vi "write_bytes.vi"(8 "error in (no error)":errorcluster, 9 "timeout ms (-1)":i32=-1, 10 "data in":string, 11 "TCP Connection in":refnum<class "TCP Connection.lvclass">) -> (0 "error out":errorcluster, 1 "bytes written":i32, 2 "timeout?":bool, 3 "TCP Connection out":refnum<class "TCP Connection.lvclass">)   [LabVIEW 2019, in "TCP Connection.lvclass"]
uses:
  TCP Connection.lvclass
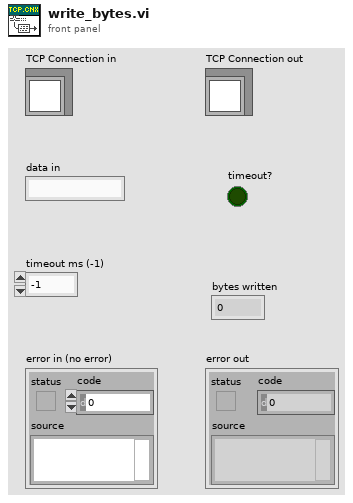
[diagram p1: front panel]
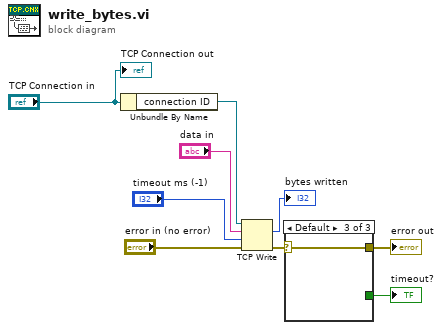
[diagram p0: block diagram]
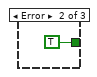
[diagram p3: hidden frame]
diagram:
  n1 = Unbundle By Name("TCP Connection in") -> ("connection ID"=w8:refnum<k5>)
  n2 = TCP Write(connection ID=w8, data in="data in", error in (no error)="error in (no error)", 9:"timeout ms (-1)") -> (bytes written=→"bytes written":i32, error out=w3:errorcluster)  [unwired: 1 out]
  n3 = case shown="Default" w3 {
    selector: w3 -> [w10 _ w12]
    tunnel: [w10 _ w12] -> w2
    tunnel: [_ TRUE _] -> w1
    frame No Error {
    }
    frame Error {
    }
    frame Default {
    }
  }
  "error out" <- w2
  "timeout?" <- w1
  "TCP Connection out" <- "TCP Connection in"
